vi "NI5112.Reset.vi"(0 "i ref in":refnum<vi>, 3 "ms timeout (100)":i32=100, 5 "error in (no error)":errorcluster) -> (14 "i ref out":refnum<vi>, 17 "timed out":bool, 19 "error out":errorcluster)   [LabVIEW 2014, in "NI5112.lvlib"]
uses:
  NI5112.lvlib
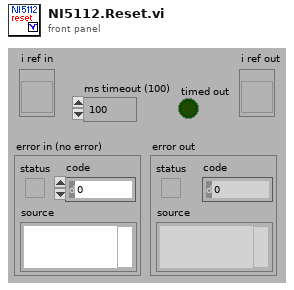
[diagram p1: front panel]
types:
  T1 = typedef "NI5112.lvlib/NI5112.i attribute.ctl" = cluster{"HWChannel":string, "instrument handle":refnum<k15>, "BinWidth":dbl, "vertical offset":dbl, "vertical range":dbl, "DataBPR":i32, "5112BPR":i32, "FullSpeed":bool, "discrLevel":dbl, "DoDiscr":bool, "VerCoupling":string}
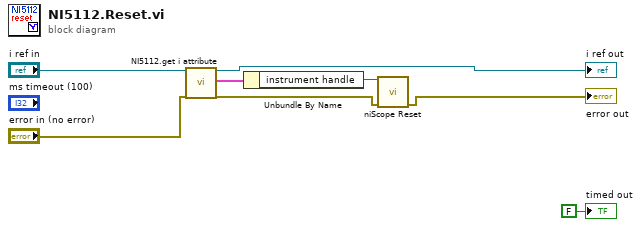
[diagram p0: block diagram]
diagram:
  n1 = call "NI5112.get i attribute.vi"("i ref in"="i ref in", "error in (no error)"="error in (no error)") -> ("i ref out"=→"i ref out":refnum<vi>, "i attribute"=w6:T1, "error out"=w4:errorcluster)  [unwired: 15 in]
  n2 = Unbundle By Name(w6) -> ("instrument handle"=w5:refnum<k15>)
  n3 = call <instrlib>:"niScope Reset.vi"("instrument handle"=w5, "error in"=w4) -> ("error out"=→"error out":errorcluster)  [unwired: 12 in, 1 out]
  "timed out" <- FALSE ("timed out")
